vi "Simple Test.vi"() -> ()   [LabVIEW 2018]
doc: "©2019\nWiebe Walstra\nwww.carya.nl"
uses:
  Impersonation/Threads.ctl
  Impersonate.lvclass
panel:
  out "read files 2":errorcluster
  in  "Boolean":bool
  out "read files":errorcluster
  out "Name 2":string
  out "Name":string
  in  "Login":enum16{"operator", "programmer", "no imp"}(ring)
  out "list files":errorcluster
  out "filenames":string[](array[string])
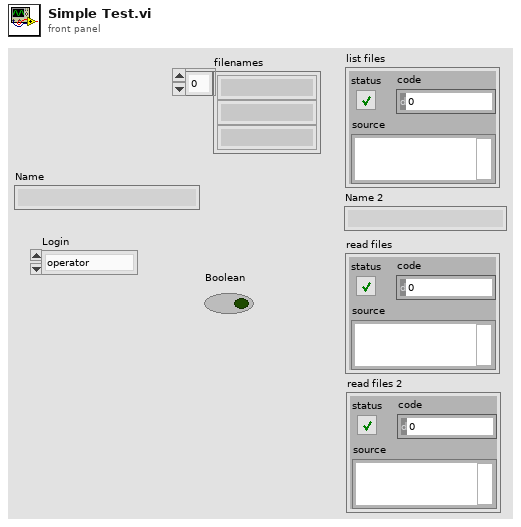
[diagram p1: front panel]
types:
  T1 = typedef "Impersonate.lvclass/Threads.ctl" = enum32{"user interface", "standard", "instrument i/o", "data acquisition", "other 1", "other 2", "same as caller", "manual"}
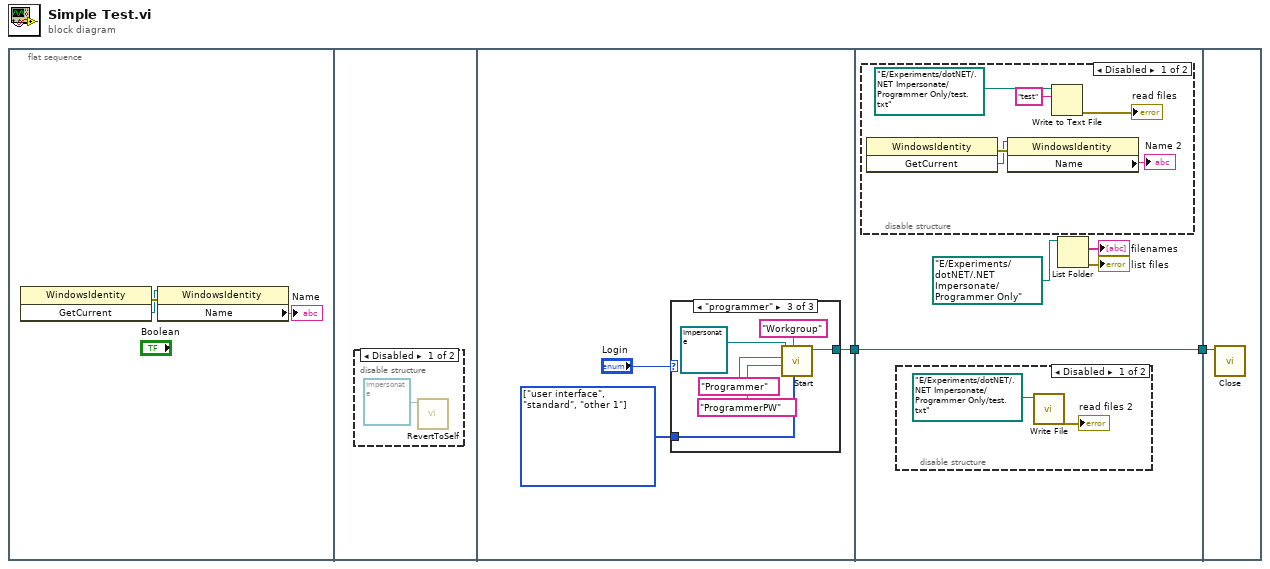
[diagram p0: block diagram]
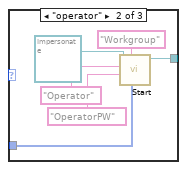
[diagram p4: hidden frame]
diagram:
  n1 = flat-sequence {
    tunnel: [w7] -> w1
    tunnel: [w23] -> w2
    tunnel: w1 -> [w23]
    tunnel: w2 -> [w34]
    frame #0 {
      n2 = invoke class="WindowsIdentity" method="GetCurrent"() -> (error out=w5:errorcluster, "GetCurrent"=w4:refnum<k24>)  [unwired: 3 in, 1 out]
      n3 = property class="WindowsIdentity"(reference=w4, error in=w5) -> ("Name"=→"Name":string)  [unwired: 2 out]
    }
    frame #1 {
      n4 = disable-structure shown="Disabled" {
        frame Disabled {
          n5 = call-dynamic "RevertToSelf.vi"("Impersonate in"=refnum<class "Impersonate.lvclass"> refnum) -> ()  [unwired: 9 in, 2 out]
        }
        frame Enabled {
        }
      }
    }
    frame #2 {
      w8 = T1[] [enum."user interface", enum."standard", enum."other 1"] items=["user interface", "standard", "instrument i/o", "data acquisition", "other 1", "other 2", "same as caller", "manual"] ("Thread")
      n6 = case shown="\"programmer\"" "Login" {
        tunnel: [_ w14 w20] -> w7
        tunnel: w8 -> [_ w10 w16]
        frame Default {
        }
        frame "operator" {
          n7 = call-dynamic "Start.vi"("Thread"=w10, "domainName"="Workgroup", "password"="OperatorPW", "userName"="Operator", "Impersonate in"=refnum<class "Impersonate.lvclass"> refnum) -> ("Impersonate out"=w14:refnum<class "Impersonate.lvclass">)  [unwired: 5 in, 1 out]
        }
        frame "programmer" {
          n8 = call-dynamic "Start.vi"("Thread"=w16, "domainName"="Workgroup", "password"="ProgrammerPW", "userName"="Programmer", "Impersonate in"=refnum<class "Impersonate.lvclass"> refnum) -> ("Impersonate out"=w20:refnum<class "Impersonate.lvclass">)  [unwired: 5 in, 1 out]
        }
      }
    }
    frame #3 {
      n9 = disable-structure shown="Disabled" {
        frame Disabled {
          n10 = invoke class="WindowsIdentity" method="GetCurrent"() -> (error out=w33:errorcluster, "GetCurrent"=w32:refnum<k24>)  [unwired: 3 in, 1 out]
          n11 = property class="WindowsIdentity"(reference=w32, error in=w33) -> ("Name"=→"Name 2":string)  [unwired: 2 out]
          n12 = Write to Text File(file (use dialog)=path "E:/Experiments/dotNET/.NET Impersonate/Programmer Only/test.txt" ("path"), text="test") -> (error out=→"read files":errorcluster)  [unwired: 2 in, 2 out]
        }
        frame Enabled {
        }
      }
      n13 = disable-structure shown="Disabled" {
        frame Disabled {
          n14 = call "Write File.vi"("path"=path "E:/Experiments/dotNET/.NET Impersonate/Programmer Only/test.txt") -> ("error out"=→"read files 2":errorcluster)  [unwired: 10 in]
        }
        frame Enabled {
        }
      }
      n15 = List Folder(path=path "E:/Experiments/dotNET/.NET Impersonate/Programmer Only") -> (filenames=→"filenames":string[], error out=→"list files":errorcluster)  [unwired: 3 in, 2 out]
    }
    frame #4 {
      n16 = call-dynamic "Close.vi"("Impersonate in"=w34) -> ()  [unwired: 9 in, 2 out]
    }
  }
